vi "Convert Pa to dBSPL.vi"(10 "Pa rms":dbl) -> (2 "dBSPL":dbl)   [LabVIEW 2022 SP3]
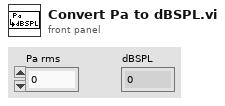
[diagram p1: front panel]
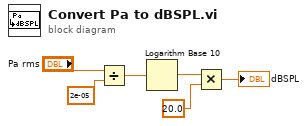
[diagram p0: block diagram]
diagram:
  n1 = Divide(x="Pa rms", y=2e-05) -> (x/y=w3:dbl)
  n2 = Logarithm Base 10(1:w3) -> (0:w4:dbl)
  n3 = Multiply(x=w4, y=20.0) -> (x*y=→"dBSPL":dbl)
